vi "VCS Set State.vi"(8 "error in (no error)":errorcluster, 9 "state":enum16{"Disabled", "Enabled", "Quickstop"}(ring), 11 "axis in":cluster{"keyHandle":u32, "nodeId":u16}={"keyHandle"=0, "nodeId"=1}) -> (0 "error out":errorcluster, 3 "axis out":cluster{"keyHandle":u32, "nodeId":u16}={"keyHandle"=0, "nodeId"=1})   [LabVIEW 2010]
doc: "<B>VCS_SetState</B> reads the actual state machine state."
uses:
  Resources/EposCmd.dll
  Resources/EposCmd64.dll
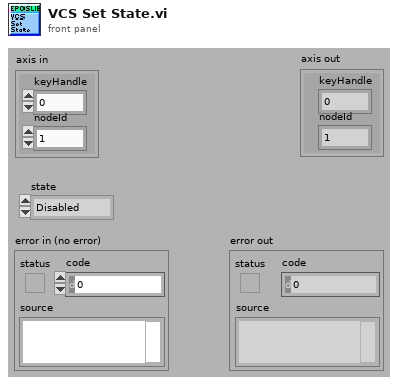
[diagram p1: front panel]
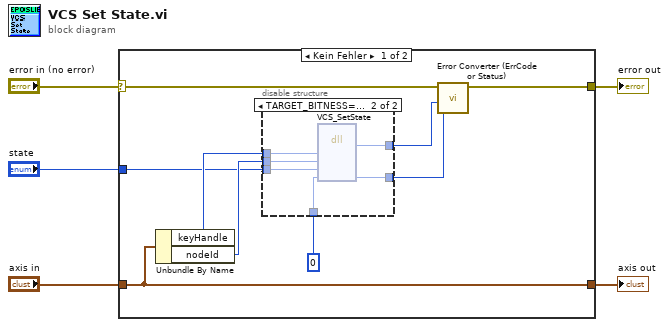
[diagram p0: block diagram]
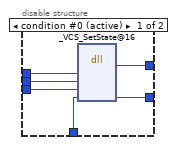
[diagram p2: hidden frame]
diagram:
  n1 = case shown="Kein Fehler" "error in (no error)" {
    selector: "error in (no error)" -> [w12 w27]
    tunnel: "axis in" -> [w14 w28]
    tunnel: [w14 w28] -> w4
    tunnel: [w13 w27] -> w3
    tunnel: "state" -> [w6 _]
    frame No Error {
      n2 = Unbundle By Name(w14) -> ("keyHandle"=w10:u32, "nodeId"=w11:u16)
      n3 = disable-structure shown="TARGET_BITNESS==64" {
        disable-tunnel: w6 -> [w20 w26]
        disable-tunnel: w11 -> [w19 w25]
        disable-tunnel: w10 -> [w18 w24]
        disable-tunnel: u32 0 ("pErrorCode") -> [w17 w23]
        disable-tunnel: [w16 w22] -> w8
        disable-tunnel: [w15 w21] -> w7
        frame condition #0 (active) {
          n4 = dll-call lib="C:/Sources/LabView/maxon EPOS/Resources/EposCmd.*" fn="_VCS_SetState@16"("KeyHandle"=w18, "NodeId"=w19, "State"=w20, "pErrorCode"=w17) -> (w15:i32, "pErrorCode"=w16:u32)  [unwired: 6 in, 2 out]
        }
        frame condition #1 {
          n5 = dll-call lib="C:/setup/Resources/EposCmd64.*" fn="VCS_SetState" ("EposCmd.dll:_VCS_SetState@16")("KeyHandle"=w24, "NodeId"=w25, "State"=w26, "pErrorCode"=w23) -> ("Rückgabetyp"=w21:i32, "pErrorCode"=w22:u32)  [unwired: 6 in, 2 out]
        }
      }
      n6 = call "Error Converter (ErrCode or Status).vi"("error code"=w8, "return type"=w7, "error in (no error)"=w12) -> ("error out"=w13:errorcluster)  [unwired: 7 in]
    }
    frame Error {
    }
  }
  "error out" <- w3
  "axis out" <- w4
